vi "Send PUBLISH.vi"(0 "WAMP Client in":refnum<class "WAMP Client.lvclass">, 5 "Message Loop Shift Register Data (In)":T2, 7 "Publish Request Data":T1, 11 "error in (no error)":errorcluster) -> (4 "WAMP Client out":refnum<class "WAMP Client.lvclass">, 6 "Message Loop Shift Register Data (Out)":T2, 15 "error out":errorcluster)   [LabVIEW 2020, in "wamplv.lvlib" / "WAMP Client.lvclass"]
uses:
  WAMP Client.lvclass
  WAMP Client.lvclass/WAMP Client.ctl
  TypeDef/PUBLISH Request Data.ctl
  TypeDef/Publish Requests Map.ctl
  API/TypeDefs/WAMP error.ctl
  TypeDef/Success or error.ctl
  TypeDef/REGISTER Request Data.ctl
  TypeDef/Message Loop Data.ctl
  TypeDef/Endpoint Data.ctl
  TypeDef/CALL Request Map.ctl
  TypeDef/EVENT payload.ctl
  TypeDef/Subscribe Result.ctl
  TypeDef/SUBSCRIBE Request Data.ctl
  TypeDef/SUBSCRIBE Requests Map.ctl
  TypeDef/Subscription Details.ctl
  TypeDef/Subscriptions Map.ctl
  TypeDef/UNSUBSCRIBE Result.ctl
  TypeDef/UNSUBSCRIBE Request Data.ctl
  TypeDef/Unsubscribe Requests Map.ctl
  API/TypeDefs/Combined error.ctl
  TypeDef/Unregister request.ctl
  TypeDef/Unregister requests map.ctl
  TypeDef/PUBLISH result.ctl
  Private/Requests/Call/ICallRequest/ICallRequest.lvclass
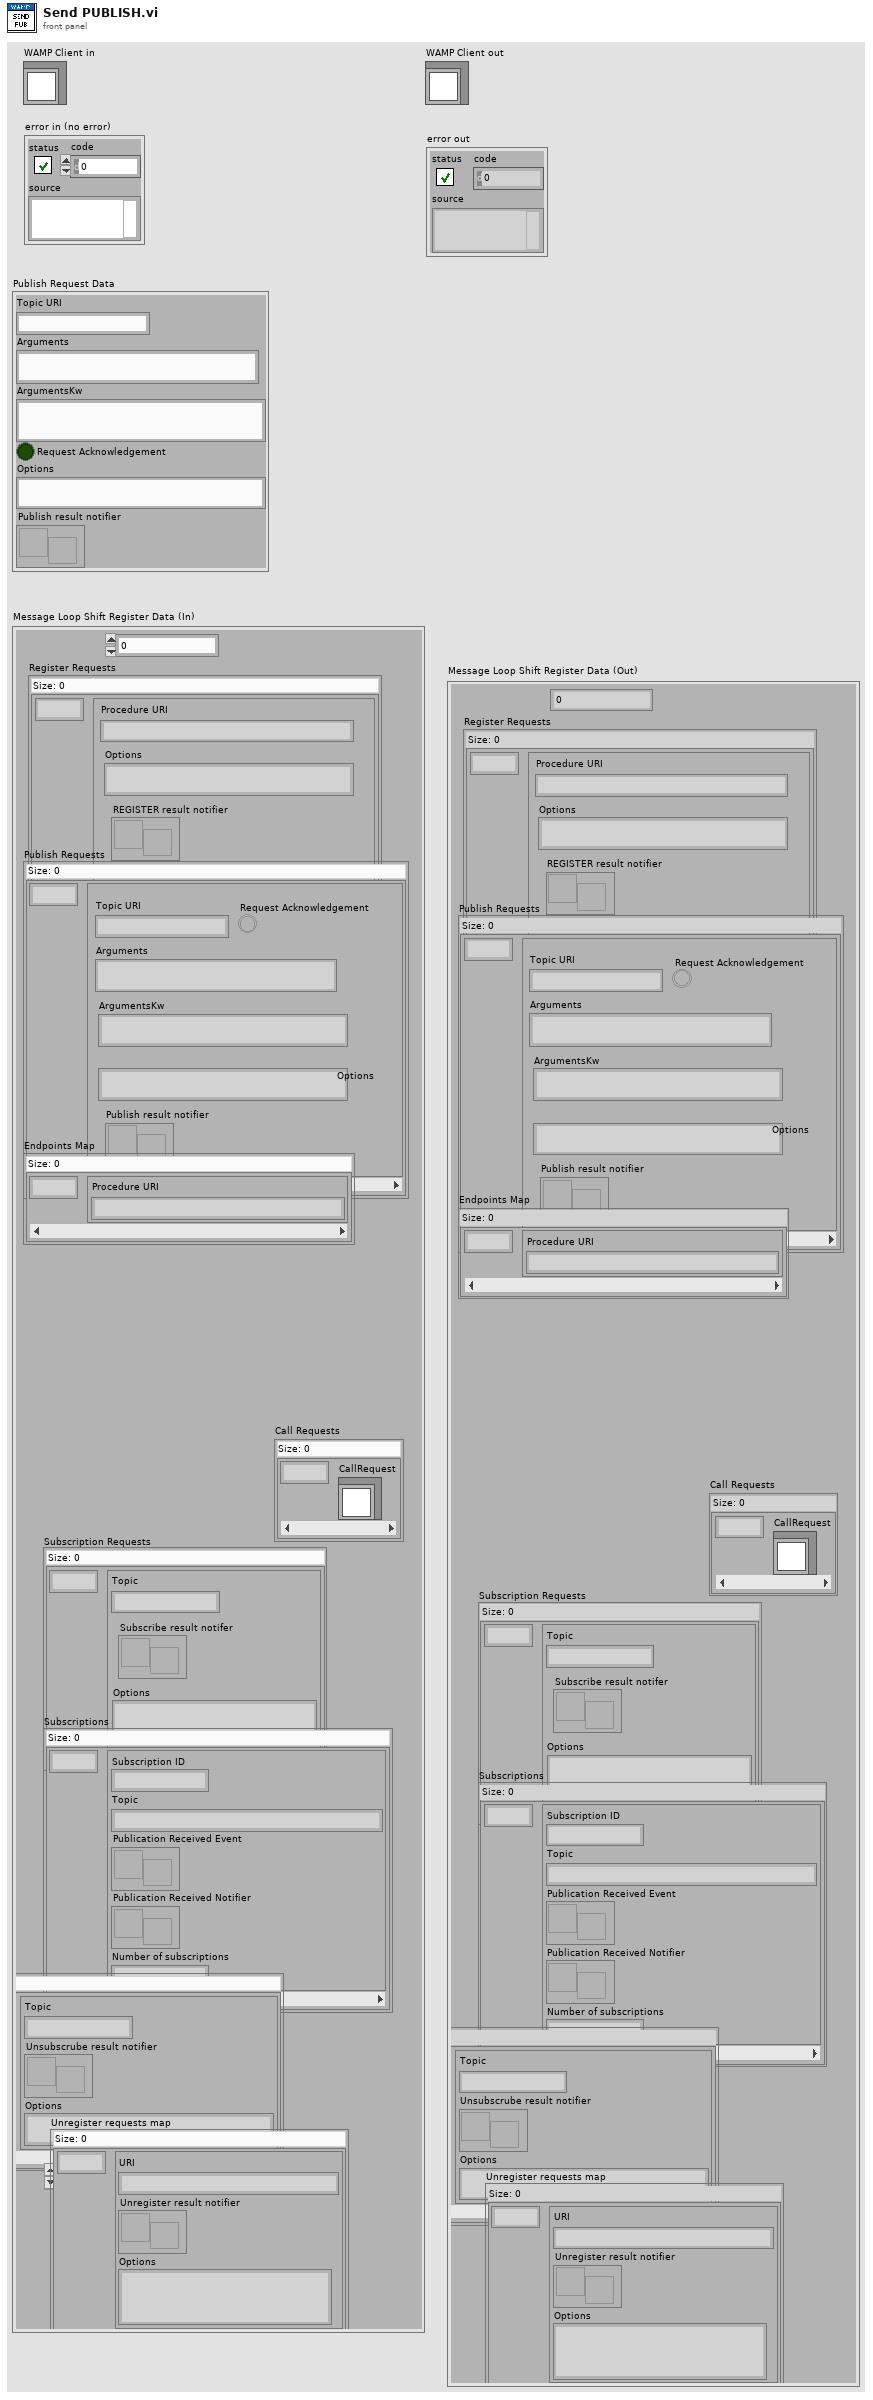
[diagram p1: front panel]
types:
  T1 = typedef "wamplv.lvlib/WAMP Client.lvclass/PUBLISH Request Data.ctl" = cluster{"Topic URI":string, "Arguments":string, "ArgumentsKw":string, "Request Acknowledgement":bool, "Options":string, "Publish result notifier":refnum<notifier>}
  T2 = typedef "wamplv.lvlib/WAMP Client.lvclass/Message Loop Data.ctl" = cluster{"Last Request ID":u64, "Register Requests":map{u64, T3}, "Publish Requests":T4, "Endpoints Map":map{u64, T5}, "Call Requests":T6, "Subscription Requests":T7, "Subscriptions":T9, "Unsubscribe Requests":T11, "Random Request IDs":u64[], "Unregister requests map":T13}
  T3 = typedef "wamplv.lvlib/WAMP Client.lvclass/REGISTER Request Data.ctl" = cluster{"Procedure URI":string, "Options":string, "REGISTER result notifier":refnum<notifier>}
  T4 = typedef "wamplv.lvlib/WAMP Client.lvclass/Publish Requests Map.ctl" = map{u64, T1}
  T5 = typedef "wamplv.lvlib/WAMP Client.lvclass/Endpoint Data.ctl" = cluster{"Procedure URI":string}
  T6 = typedef "wamplv.lvlib/WAMP Client.lvclass/CALL Request Map.ctl" = map{u64, refnum<class "ICallRequest.lvclass">}
  T7 = typedef "wamplv.lvlib/WAMP Client.lvclass/SUBSCRIBE Requests Map.ctl" = map{u64, T8}
  T8 = typedef "wamplv.lvlib/WAMP Client.lvclass/SUBSCRIBE Request Data.ctl" = cluster{"Topic":string, "Subscribe result notifer":refnum<notifier>, "Options":string}
  T9 = typedef "wamplv.lvlib/WAMP Client.lvclass/Subscriptions Map.ctl" = map{u64, T10}
  T10 = typedef "wamplv.lvlib/WAMP Client.lvclass/Subscription Details.ctl" = cluster{"Subscription ID":u64, "Topic":string, "Publication Received Event":refnum<user-event>, "Publication Received Notifier":refnum<notifier>, "Number of subscriptions":u64}
  T11 = typedef "wamplv.lvlib/WAMP Client.lvclass/Unsubscribe Requests Map.ctl" = map{u64, T12}
  T12 = typedef "wamplv.lvlib/WAMP Client.lvclass/UNSUBSCRIBE Request Data.ctl" = cluster{"Topic":string, "Unsubscrube result notifier":refnum<notifier>, "Options":string}
  T13 = typedef "wamplv.lvlib/WAMP Client.lvclass/Unregister requests map.ctl" = map{u64, T14}
  T14 = typedef "wamplv.lvlib/WAMP Client.lvclass/Unregister request.ctl" = cluster{"URI":string, "Unregister result notifier":refnum<notifier>, "Options":string}
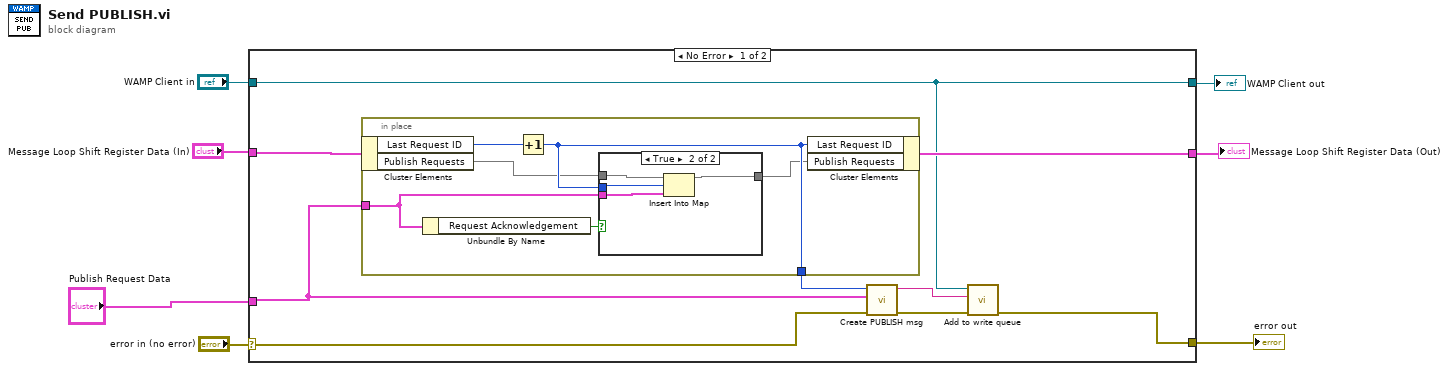
[diagram p0: block diagram]
diagram:
  n1 = case shown="No Error" "error in (no error)" {
    selector: "error in (no error)" -> [w16 w30]
    tunnel: [w8 w30] -> w6
    tunnel: [w10 w29] -> w4
    tunnel: "WAMP Client in" -> [w10 w29]
    tunnel: "Publish Request Data" -> [w15 _]
    tunnel: "Message Loop Shift Register Data (In)" -> [w13 w28]
    tunnel: [w12 w28] -> w2
    frame No Error {
      n2 = in-place "In Place Element Structure" {
        in-place-border: w15 -> [w21]
        in-place-border: [w19] -> w14
        n3 = in-place-cluster #1(w13) -> ("Last Request ID"=w20:u64, "Publish Requests"=w17:T4)
        n4 = Unbundle By Name(w21) -> ("Request Acknowledgement"=w22:bool)
        n5 = Increment(x=w20) -> (x+1=w19:u64)
        n6 = case shown="True" w22 {
          tunnel: w17 -> [w23 w27]
          tunnel: w21 -> [_ w26]
          tunnel: [w23 w25] -> w18
          tunnel: w19 -> [_ w24]
          frame False {
          }
          frame True {
            n7 = Insert Into Map(map in=w27, key=w24, value=w26) -> (map out=w25:T4)  [unwired: 2 out]
          }
        }
        n8 = in-place-cluster #1("Last Request ID"=w19, "Publish Requests"=w18) -> (w12:T2)
      }
      n9 = call "Create PUBLISH msg.vi"("error in"=w16, "Publish Requst"=w15, "Request ID"=w14) -> ("error out"=w11:errorcluster, "WAMP Message"=w9:string)  [unwired: 7 in]
      n10 = call "Add to write queue.vi"("error in (no error)"=w11, "Write item"=w9, "WAMP Client in"=w10) -> ("error out"=w8:errorcluster)  [unwired: 8 in]
    }
    frame Error {
    }
  }
  "error out" <- w6
  "WAMP Client out" <- w4
  "Message Loop Shift Register Data (Out)" <- w2
